vi "TR_Load_raw_data_from_TDMS.vi"(8 "error in (no error)":errorcluster, 9 "Decimate?":bool, 10 "Defragment TDMS? (F)":bool, 11 "TDMS track ref. in":path) -> (0 "error out":errorcluster, 1 "SW timestamp":dbl[](array[numeric]), 2 "HW ts and Frame HW time":u32[][](array[numeric]), 3 "TDMS track ref. out":refnum<k34>, 4 "TTL IO and Key":string[][](array[string]), 5 "Raw values":dbl[][](array[numeric]))   [LabVIEW 2018, in "Tracks Repair.lvlib"]
uses:
  Tracks Repair.lvlib
  52988af9-cea8-4ca2-8122-a15f69f19891.vi
  9b366c35-48b3-4647-a9a0-5904c1a5bb15.vi
  3d8eb5a0-8714-431c-bea7-f6ba7842037e.vi
  b12873a5-3919-43b5-b92e-eb58822e0316.vi
  52988af9-cea8-4ca2-8122-a15f69f19891.vi/4c0c65f7-7a95-43c8-8d56-9335e06c2918.vi
  9b366c35-48b3-4647-a9a0-5904c1a5bb15.vi/24962e30-4e89-41fb-9a19-e399aa91a2c0.vi
  3d8eb5a0-8714-431c-bea7-f6ba7842037e.vi/bc598129-7384-4d20-b801-8b01f419b6ba.vi
  b12873a5-3919-43b5-b92e-eb58822e0316.vi/ccc63096-44e8-44af-880f-48bca0cb5b0e.vi
  <vilib>/Utility/Data Type/Get Type Information.vi
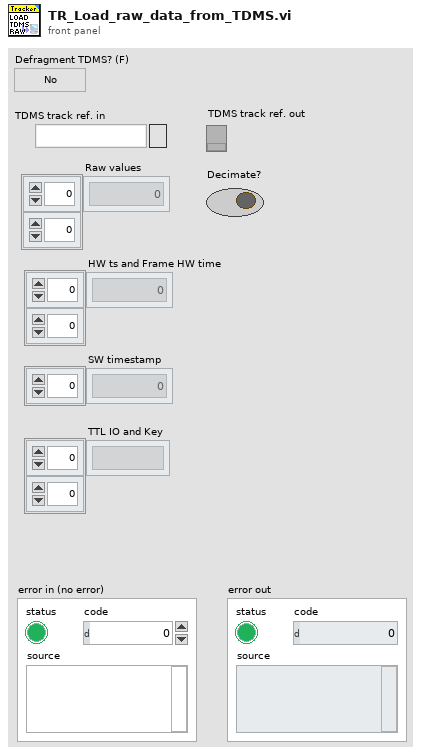
[diagram p1: front panel]
types:
  T1 = enum16{"big-endian, network order", "native, host order", "little-endian"}
  T2 = enum16{"open", "open or create", "create or replace", "create", "open (read-only)"}
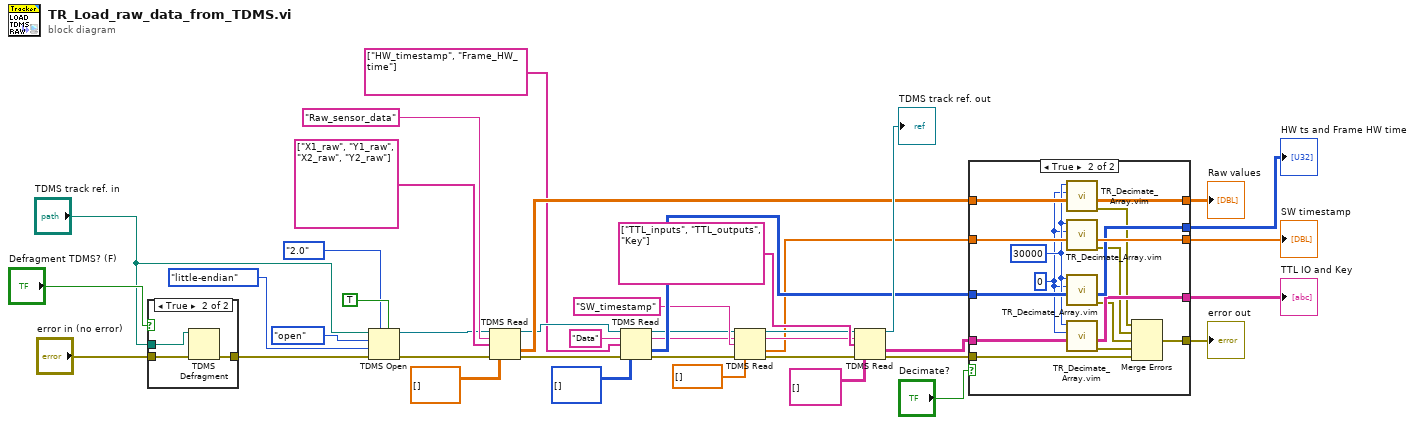
[diagram p0: block diagram]
diagram:
  n1 = case shown="True" "Defragment TDMS? (F)" {
    tunnel: "TDMS track ref. in" -> [_ w44]
    tunnel: "error in (no error)" -> [w41 w43]
    tunnel: [w41 w42] -> w13
    frame False {
    }
    frame True {
      n2 = TDMS Defragment(4:w43, 7:w44) -> (0:w42:errorcluster)
    }
  }
  n3 = TDMS Open(5:TRUE ("create index file? (T)"), 7:enum16{"1.0", "2.0"}."2.0" ("file format version (2.0)"), 8:w13, 9:T1."little-endian" ("byte order (2:little-endian)"), 10:T2."open" ("operation (0:open)"), 11:"TDMS track ref. in") -> (0:w9:errorcluster, 3:w16:refnum<k34>)  [unwired: 1 in]
  n4 = TDMS Read(0:w16, 5:"Raw_sensor_data" ("group name"), 7:string[] ["X1_raw", "Y1_raw", "X2_raw", "Y2_raw"] ("Columns Names"), 11:w9, 12:dbl[][] [] ("appended array")) -> (4:w28:refnum<k34>, 10:w29:dbl[][], 15:w40:errorcluster)  [unwired: 3 in, 3 out]
  n5 = TDMS Read(0:w28, 5:"Data" ("group name in"), 7:string[] ["HW_timestamp", "Frame_HW_time"] ("appended array"), 11:w40, 12:u32[][] [] ("appended array")) -> (4:w25:refnum<k34>, 6:w24:string, 10:w30:u32[][], 15:w23:errorcluster)  [unwired: 3 in, 2 out]
  n6 = TDMS Read(0:w25, 5:w24, 7:"SW_timestamp" ("channel name(s) in (Untitled)"), 11:w23, 12:dbl[] [] ("appended array")) -> (4:w33:refnum<k34>, 6:w36:string, 10:w2:dbl[], 15:w34:errorcluster)  [unwired: 3 in, 2 out]
  n7 = TDMS Read(0:w33, 5:w36, 7:string[] ["TTL_inputs", "TTL_outputs", "Key"] ("channel name(s) in (Untitled)"), 11:w34, 12:string[][] [] ("appended array")) -> (4:→"TDMS track ref. out":refnum<k34>, 10:w39:string[][], 15:w3:errorcluster)  [unwired: 3 in, 3 out]
  n8 = case shown="True" "Decimate?" {
    tunnel: w39 -> [w46 w56]
    tunnel: w30 -> [w48 w60]
    tunnel: w29 -> [w49 w63]
    tunnel: w2 -> [w47 w62]
    tunnel: [w49 w65] -> w8
    tunnel: [w48 w59] -> w7
    tunnel: [w47 w61] -> w6
    tunnel: [w46 w55] -> w5
    tunnel: w3 -> [w45 w64]
    tunnel: [w45 w54] -> w1
    frame False {
    }
    frame True {
      w57 = 0 ("Offset")
      w58 = 30000 ("Target length")
      n9 = call "TR_Decimate_Array.vim"("Array in"=w63, "Offset"=w57, "Target length"=w58) -> ("error out"=w53:errorcluster, "Array out"=w65:dbl[][])  [unwired: 7 in]
      n10 = call "TR_Decimate_Array.vim"("Array in"=w62, "Offset"=w57, "Target length"=w58) -> ("error out"=w52:errorcluster, "Array out"=w61:dbl[])  [unwired: 7 in]
      n11 = call "TR_Decimate_Array.vim"("Array in"=w60, "Offset"=w57, "Target length"=w58) -> ("error out"=w51:errorcluster, "Array out"=w59:u32[][])  [unwired: 7 in]
      n12 = call "TR_Decimate_Array.vim"("Array in"=w56, "Offset"=w57, "Target length"=w58) -> ("error out"=w50:errorcluster, "Array out"=w55:string[][])  [unwired: 7 in]
      n13 = Merge Errors(w53, w52, w51, w50, w64) -> (w54:errorcluster)
    }
  }
  "error out" <- w1
  "Raw values" <- w8
  "HW ts and Frame HW time" <- w7
  "SW timestamp" <- w6
  "TTL IO and Key" <- w5
